vi "Calculate Sample Rate.vi"(0 "Register Bus":T1, 5 "sample rate [S/s]":dbl=10000000.0 min=1.0 max=250000000.0 format="%#.3pS/s", 11 "error in":errorcluster) -> (4 "Register Bus (out)":T1, 6 "sample rate [ratio]":dbl, 15 "error out":errorcluster)   [LabVIEW 2017]
doc: "Calculate the sample rate value to write to the device's DSP blocks.\n\n<B>Input Parameters</B>\n\n<B>Register Bus</B> The Register Bus object created by the ni579x Open VI and used as the session handle for the NI-579x Configuration Design Library.\n\n<B>sample rate [S/s]</B> is the requested sample rate (in samples per second).\n\n<B>error in</B> describes error conditions that occur before this node runs. This input provides standard 'error in' functionality.\n\n<B>Output Parameters</B>\n\n<B>Register Bus (out)</B> The Register Bus object created by the ni579x Open VI and used as the session handle for the NI-579x Configuration Design Library.\n\n<B>sample rate [ratio]</B> is the value to write to the device's DSP blocks.\n\n<B>error out</B> contains error information. This output provides standard 'error out' functionality."
uses:
  <instrlib>/_niInstr/Register Bus/v0/Host/Public/Register Bus Session.ctl
  <instrlib>/_niInstr/Register Bus/v0/Host/Private/Session Data.ctl
  <vilib>/Utility/error.llb/Error Cluster From Error Code.vi
  <vilib>/ErrorRing/Error Ring.xnode
  <instrlib>/ni579x/Config/v2/Host/ni579x Config v2 Host.lvlib
  <instrlib>/_niInstr/Register Bus/v0/Host/niInstr Register Bus v0 Host.lvlib
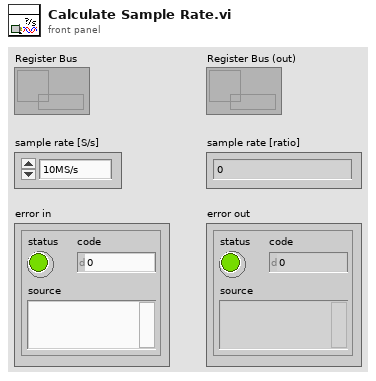
[diagram p1: front panel]
types:
  T1 = typedef "niInstr Register Bus v0 Host.lvlib/Register Bus Session.ctl" = refnum<queue>
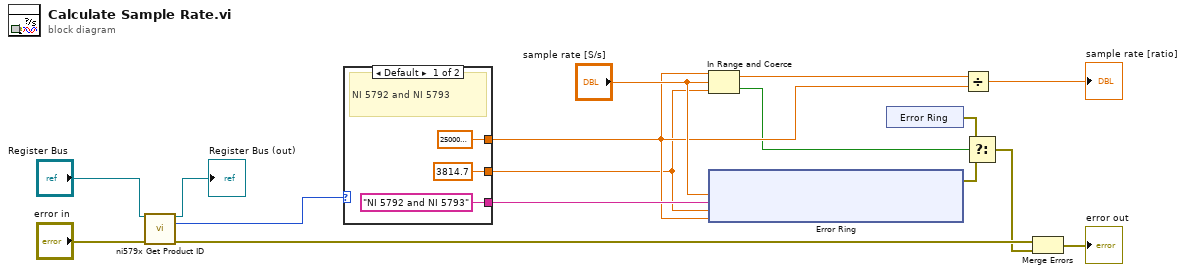
[diagram p0: block diagram]
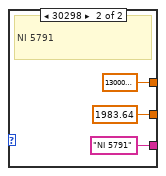
[diagram p2: hidden frame]
diagram:
  n1 = call <instrlib>:"ni579x Get Product ID.vi"("Register Bus"="Register Bus", "Error In"="error in") -> ("Register Bus (out)"=→"Register Bus (out)":T1, "product ID"=w12:u16, "Error Out"=w7:errorcluster)  [unwired: 11 in]
  n2 = case shown="Default" w12 {
    tunnel: [250000000.0 ("clock rate [Hz]") 130000000.0 ("clock rate [Hz]")] -> w9
    tunnel: ["NI 5792 and NI 5793" "NI 5791"] -> w10
    tunnel: [3814.7 ("lower limit") 1983.64 ("lower limit")] -> w1
    frame Default {
      # "NI 5792 and NI 5793"
    }
    frame 30298 {
      # "NI 5791"
    }
  }
  n3 = In Range and Coerce(upper limit=w9, x="sample rate [S/s]", lower limit=w1) -> (coerced(x)=w16:dbl, In Range?=w8:bool)
  n4 = xnode ("Error Ring")("parameter 0"="sample rate [S/s]", "parameter 1"=w10, "parameter 2"=w1, "parameter 3"=w9) -> ("error out"=w4:errorcluster)
  n5 = xnode ("Error Ring")() -> ("error out"=w3:errorcluster)
  n6 = Divide(x=w16, y=w9) -> (x/y=→"sample rate [ratio]":dbl)
  n7 = Select(t=w3, s=w8, f=w4) -> (s? t:f=w6:errorcluster)
  n8 = Merge Errors(w7, w6) -> (→"error out":errorcluster)
